vi "Insert Guide Point.vi"(8 "error in (no error)":errorcluster, 11 "Channel in":refnum<class "Channel.lvclass">) -> (0 "error out":errorcluster, 3 "Channel out":refnum<class "Channel.lvclass">)   [LabVIEW 2018, in "Channel.lvclass"]
uses:
  Channel.lvclass
  Channel.lvclass/Channel.ctl
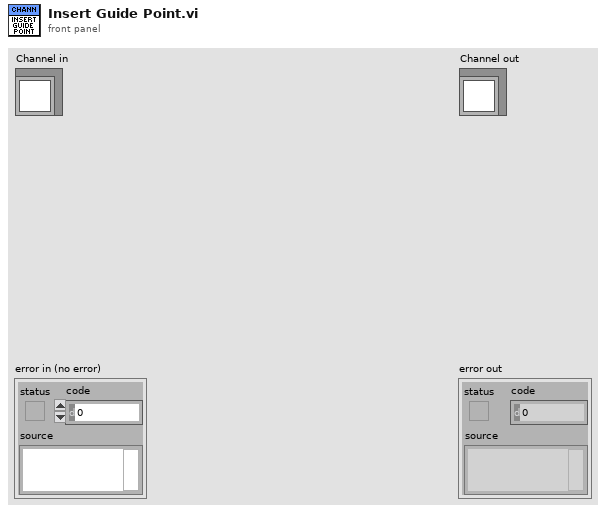
[diagram p1: front panel]
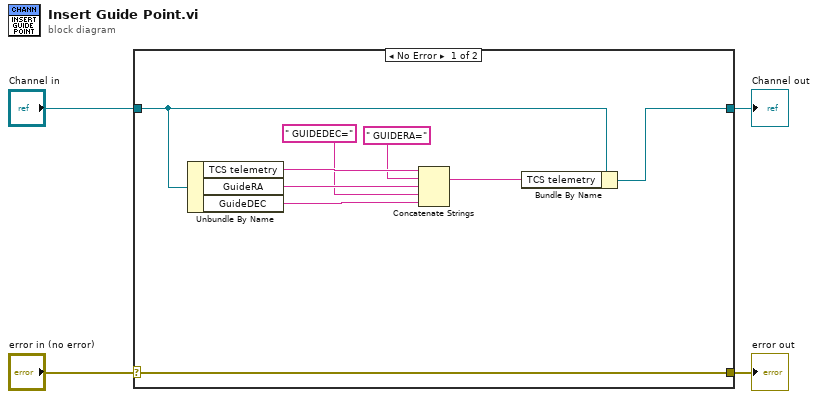
[diagram p0: block diagram]
diagram:
  n1 = case shown="No Error" "error in (no error)" {
    selector: "error in (no error)" -> [w13 w15]
    tunnel: [w13 w15] -> w3
    tunnel: [w5 w14] -> w1
    tunnel: "Channel in" -> [w7 w14]
    frame No Error {
      n2 = Unbundle By Name(w7) -> ("TCS telemetry"=w12:string, "GuideRA"=w10:string, "GuideDEC"=w8:string)
      n3 = Concatenate Strings(w12, " GUIDERA=" ("string"), w10, " GUIDEDEC=" ("string"), w8) -> (w6:string)
      n4 = Bundle By Name(cluster=w7, "TCS telemetry"=w6) -> (w5:refnum<class "Channel.lvclass">)
    }
    frame Error {
    }
  }
  "error out" <- w3
  "Channel out" <- w1
